vi "MainTest(Elapsed Timer).vi"() -> ()   [LabVIEW 2018]
panel:
  in  "stop":bool
  in  "Press to Pause":bool
  out "Elapsed time":dbl=3.054077625274658 format="%#.2g"
  out "Flag":bool
  out "Paused timer":bool
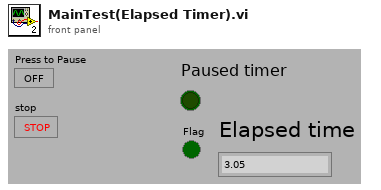
[diagram p1: front panel]
types:
  T1 = enum16{"Init Timer", "Start Timer", "Paused Timer"}
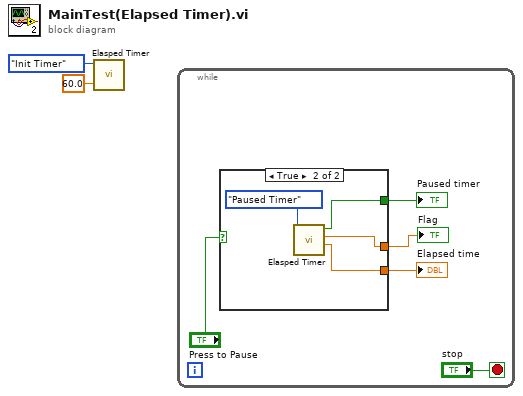
[diagram p0: block diagram]
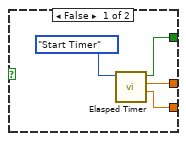
[diagram p2: hidden frame]
diagram:
  n1 = call "Elasped Timer.vi"("Time Setting"=60.0 ("set time"), "Action"=T1."Init Timer" ("states")) -> ()  [unwired: 6 in, 4 out]
  n2 = while {
    stop <- "stop" stop-if-true
    n3 = case shown="True" "Press to Pause" {
      tunnel: [w10 w15] -> w7
      tunnel: [w9 w14] -> w6
      tunnel: [w8 w13] -> w5
      frame False {
        n4 = call "Elasped Timer.vi"("Action"=T1."Start Timer" ("states")) -> ("Elapsed Time"=w8:dbl, "Time Left"=w9:dbl, "Time Out?!"=w10:bool)  [unwired: 7 in, 1 out]
      }
      frame True {
        n5 = call "Elasped Timer.vi"("Action"=T1."Paused Timer" ("states")) -> ("Elapsed Time"=w13:dbl, "Time Left"=w14:dbl, "Time Out?!"=w15:bool)  [unwired: 7 in, 1 out]
      }
    }
    "Paused timer" <- w7
    "Flag" <- w6
    "Elapsed time" <- w5
  }
